vi "Write Multiple Coil.vi"(8 "error in (no error)":errorcluster, 9 "coils to write":bool[](array[boolean]), 10 "starting address":u16, 11 "Modbus TCP in":refnum<class "Modbus TCP.lvclass">) -> (0 "error out":errorcluster, 3 "Modbus TCP out":refnum<class "Modbus TCP.lvclass">)   [LabVIEW 2023, in "HardwareAbstractionLayer_LVOOP.lvlib" / "Modbus TCP.lvclass"]
uses:
  Modbus TCP.lvclass
  Modbus TCP.lvclass/Modbus TCP.ctl
  <vilib>/NI/Modbus Library/API/Master/Modbus Master.lvclass
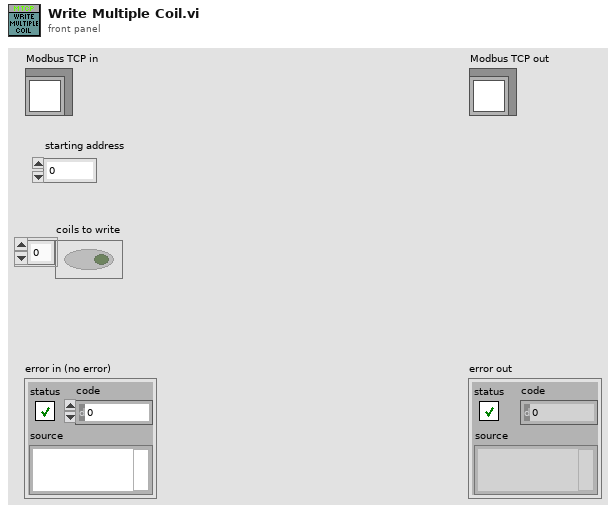
[diagram p1: front panel]
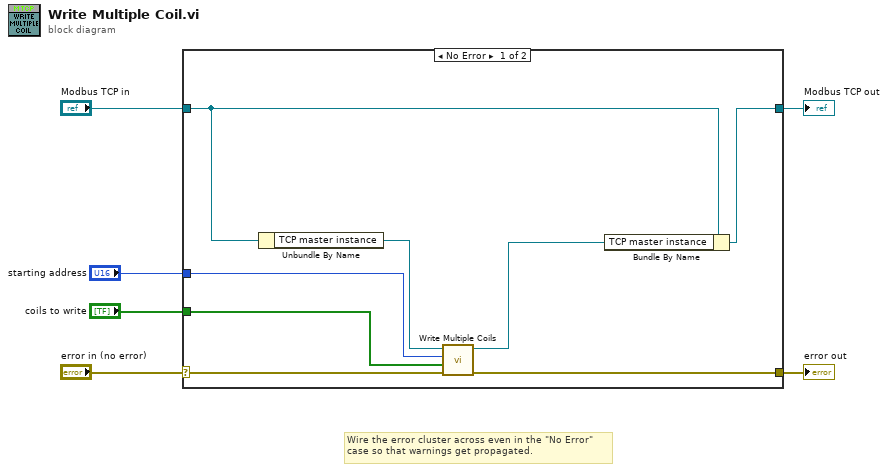
[diagram p0: block diagram]
diagram:
  # "Wire the error cluster across even in the \"No Error\"\ncase so that warnings get propagated."
  n1 = case shown="No Error" "error in (no error)" {
    selector: "error in (no error)" -> [w13 w16]
    tunnel: [w12 w16] -> w5
    tunnel: [w10 w15] -> w3
    tunnel: "Modbus TCP in" -> [w11 w15]
    tunnel: "starting address" -> [w8 _]
    tunnel: "coils to write" -> [w7 _]
    frame No Error {
      n2 = Unbundle By Name(w11) -> ("TCP master instance"=w14:refnum<class "Modbus Master.lvclass">)
      n3 = call-dynamic "Write Multiple Coils.vi"("error in"=w13, "coils to write"=w7, "starting address"=w8, "Modbus master in"=w14) -> ("error out"=w12:errorcluster, "Modbus master out"=w9:refnum<class "Modbus Master.lvclass">)  [unwired: 6 in]
      n4 = Bundle By Name(cluster=w11, "TCP master instance"=w9) -> (w10:refnum<class "Modbus TCP.lvclass">)
    }
    frame Error {
    }
  }
  "error out" <- w5
  "Modbus TCP out" <- w3
